vi "getEventForceActuatorTest.vi"(11 "UserEvents in":refnum<class "UserEvents.lvclass">) -> (2 "EventForceActuatorTest":refnum<user-event>, 3 "UserEvents out":refnum<class "UserEvents.lvclass">)   [LabVIEW 2016, in "UserEvents.lvclass"]
uses:
  UserEvents.lvclass
  DataTypes/Topics/EventForceActuatorTest.ctl
  DataTypes/Topics/Parts/Timestamp.ctl
  DataTypes/Topics/Parts/TestStatus.ctl
  UserEvents.lvclass/UserEvents.ctl
  DataTypes/Topics/M1M3SupportTopics.lvlib
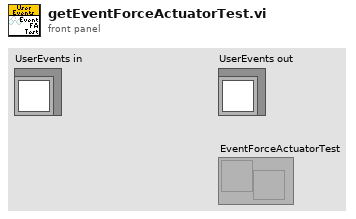
[diagram p1: front panel]
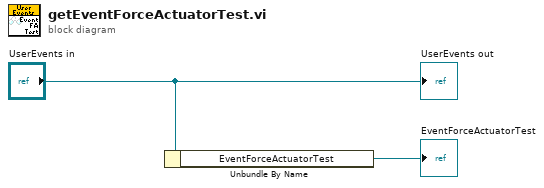
[diagram p0: block diagram]
diagram:
  n1 = Unbundle By Name("UserEvents in") -> ("EventForceActuatorTest"=→"EventForceActuatorTest":refnum<user-event>)
  "UserEvents out" <- "UserEvents in"
